vi "Untitled 1.vi"() -> ()   [LabVIEW 2019]
panel:
  out "circle info":dbl[][](array[numeric])
  out "error out":errorcluster
  out "pellet detected?":bool
  out "Image":T1(plugin-control)
  in  "function name":string="get_circels"
  in  "module path":path
  in  "Stop (F)":bool
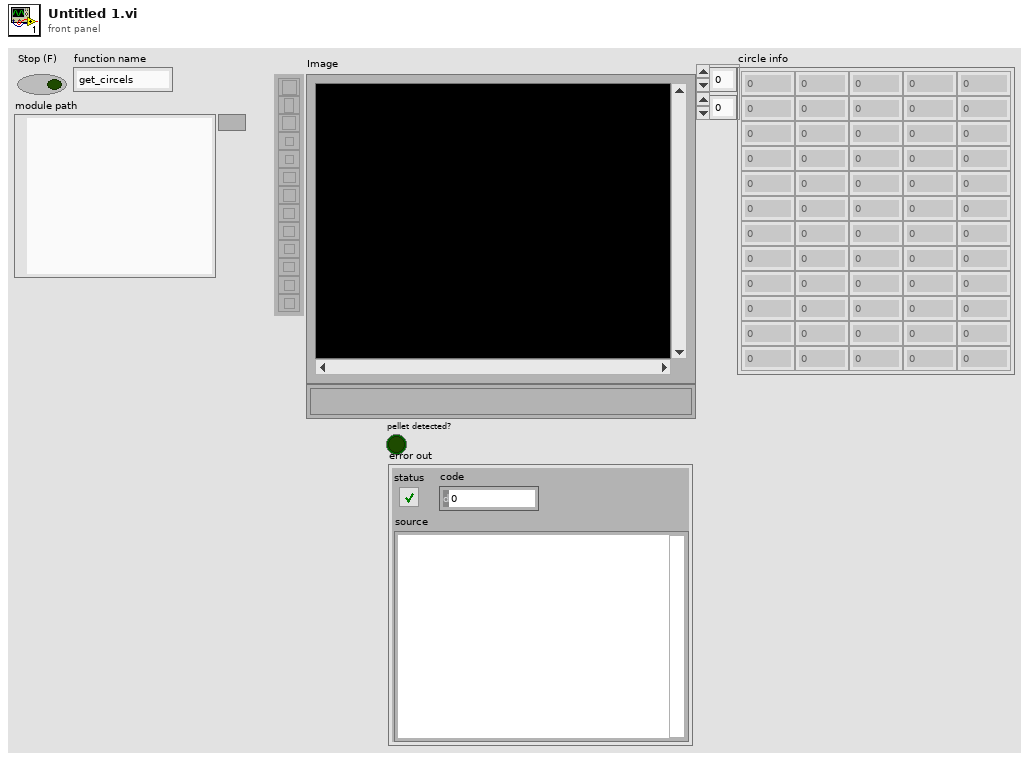
[diagram p1: front panel]
types:
  T1 = typedef "IMAQ Image.ctl" = refnum<image>
  T2 = typedef "Image Type" = u32
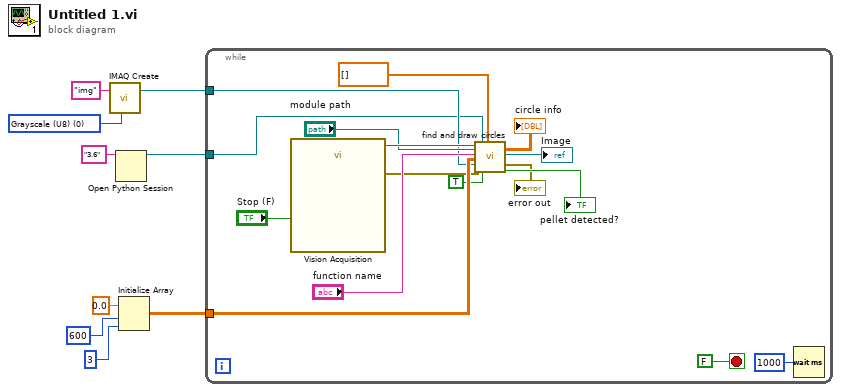
[diagram p0: block diagram]
diagram:
  w4 = T2 0 items=["Grayscale (U8)", "Grayscale (I16)", "Grayscale (SGL)", "Complex (CSG)", "RGB (U32)", "HSL (U32)", "RGB (U64)", "Grayscale (U16)"] ("Image Type")
  n1 = call "IMAQ Create"("Image Name"="img", "Image Type"=w4) -> ("New Image"=w3:T1)  [unwired: 3 in, 1 out]
  n2 = Open Python Session(python version="3.6" ("Python version")) -> (session out=w1:refnum<k35>)  [unwired: 2 in, 1 out]
  n3 = Initialize Array(0.0 ("element"), 600 ("dimension size"), 3 ("dimension size")) -> (w6:dbl[][])
  n4 = while {
    tunnel: w3 -> [w18]
    tunnel: w6 -> [w19]
    tunnel: w1 -> [w16]
    stop <- FALSE stop-if-true
    n5 = call "Vision Acquisition"("Stop (F)"="Stop (F)") -> ("Image Out"=w22:T1, "error out"=w17:errorcluster)  [unwired: 24 in, 1 out]
    n6 = call "find and draw circles.vi"("Image Src"=w22, "module path"="module path", "function name"="function name", "initialized array"=w19, "Image Dst"=w18, "error in (no error)"=w17, "session in"=w16, "Run/Stop"=TRUE, "grading Thr"=dbl[] []) -> ("circle info"=→"circle info":dbl[][], "Image Out"=→"Image":T1, "error out"=→"error out":errorcluster, "pellet detected?"=→"pellet detected?":bool)  [unwired: 6 in, 1 out]
    n7 = Wait (ms)(milliseconds to wait=u32 1000) -> ()  [unwired: 1 out]
  }
